vi "get index type definitions.vi"(11 "fixed channel configuration in":refnum<class "control module configuration.lvclass">) -> (2 "index type defs":T1, 3 "fixed channel configuration out":refnum<class "control module configuration.lvclass">)   [LabVIEW 2013, in "control module configuration.lvclass"]
uses:
  control module configuration.lvclass
  index type definitions.ctl
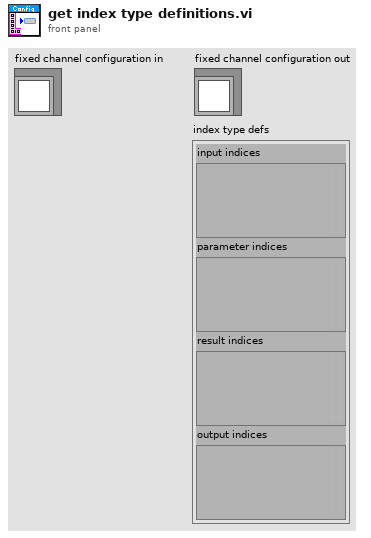
[diagram p1: front panel]
types:
  T1 = typedef "control module configuration.lvclass/index type definitions.ctl" = cluster{"input indices":variant, "parameter indices":variant, "result indices":variant, "output indices":variant}
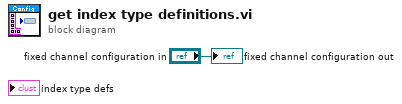
[diagram p0: block diagram]
diagram:
  "fixed channel configuration out" <- "fixed channel configuration in"
